vi "Stop Iterate.vi"(8 "error in (no error)":errorcluster, 11 "Iterator Actor in":refnum<class "Iterator Actor.lvclass">) -> (0 "error out":errorcluster, 3 "Iterator Actor out":refnum<class "Iterator Actor.lvclass">)   [LabVIEW 2016, in "Iterator Actor.lvlib" / "Iterator Actor.lvclass"]
doc: "Stops all the subsequent iterations."
uses:
  Iterator Actor.lvclass
  Iterator Actor.lvclass/Iterator Actor.ctl
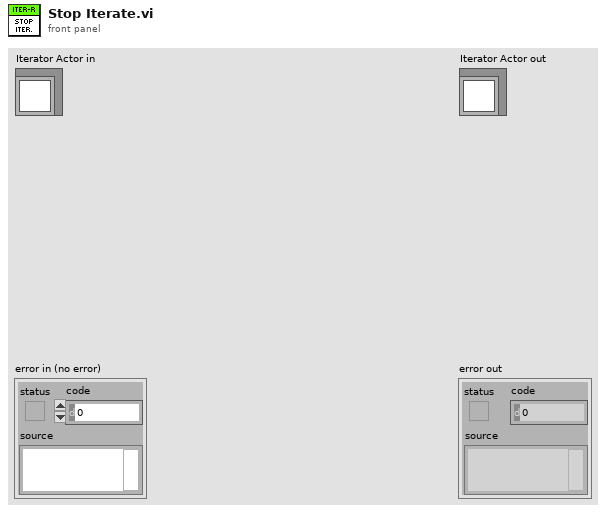
[diagram p1: front panel]
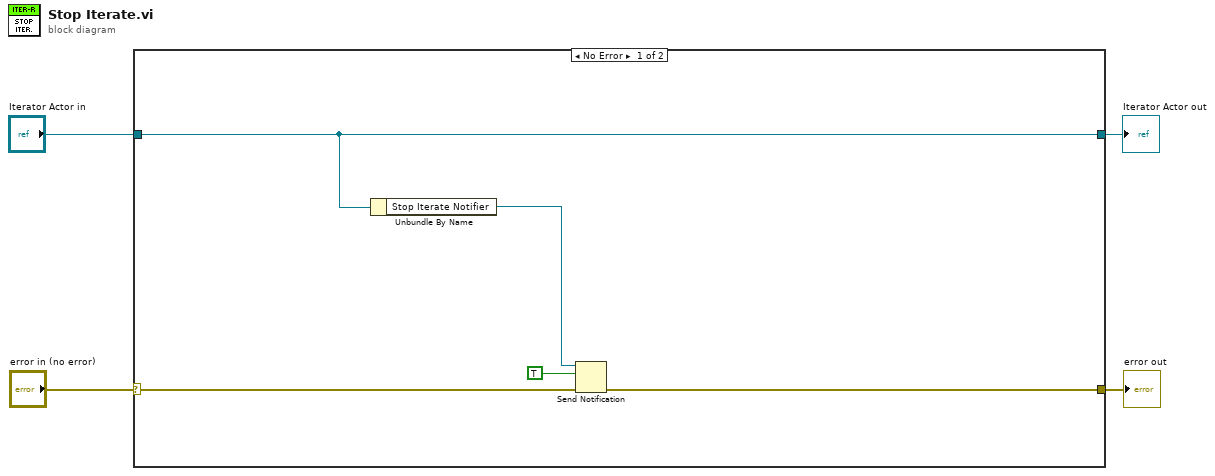
[diagram p0: block diagram]
diagram:
  n1 = case shown="No Error" "error in (no error)" {
    selector: "error in (no error)" -> [w7 w11]
    tunnel: [w8 w11] -> w3
    tunnel: [w9 w10] -> w1
    tunnel: "Iterator Actor in" -> [w9 w10]
    frame No Error {
      n2 = Unbundle By Name(w9) -> ("Stop Iterate Notifier"=w6:refnum<notifier>)
      n3 = Send Notification(notification=TRUE, notifier=w6, error in (no error)=w7) -> (error out=w8:errorcluster)  [unwired: 1 out]
    }
    frame Error {
    }
  }
  "error out" <- w3
  "Iterator Actor out" <- w1
